vi "09-QNET_MECHKIT_Encoder.vi"() -> ()   [LabVIEW 2012]
doc: "This VI is to be used with the NI-ELVIS and the QNET-Mechatronic Sensors I module. The objective is learn about the behaviour of encoders."
uses:
  <vilib>/Simulation/Scripting/Companion Diagram/SimConfigNode/SimParams.ctl
  <vilib>/Simulation/Scripting/Companion Diagram/SimConfigNode/_simSolvers.ctl
  <vilib>/Simulation/Implementation/Shared/SIMSCR Execution Mode.ctl
  <vilib>/Simulation/Param Hierarchy/Typedefs/SIMPH Param Control Actions.ctl
  <vilib>/Simulation/Implementation/Shared/NILVSim_ParamChanged.vi
  <vilib>/Simulation/SignalDisplay/Implementation/NILVSim Time Waveform.llb/SIM Time Waveform (vector).vi
  <vilib>/Simulation/Utility/Implementation/SIM Halt.vi
  <vilib>/Simulation/SignalDisplay/Implementation/NILVSim Time Waveform.llb/SIM Time Waveform (scalar).vi
  <vilib>/Simulation/Implementation/Shared/NILVSim_Manager.vi
  <vilib>/Simulation/Implementation/Shared/NILVSim_FinalizeModel.vi
  <vilib>/Simulation/Implementation/Shared/SIM Unbundle Sim Info.vi
  <vilib>/Utility/error.llb/Clear Errors.vi
  <vilib>/Simulation/Implementation/Shared/NILVSim_GetModelError.vi
  <vilib>/Simulation/Implementation/Shared/SIM Bundle Sim Info.vi
  <vilib>/Simulation/Implementation/Shared/SIMSH Read Queue.vi
  <vilib>/Simulation/Implementation/Shared/NILVSim_Initialize.vi
  QNET Library/QNET_Drivers.llb/QNET_MECHKIT_AI_Read.vi
  <vilib>/Simulation/Utility/Implementation/NILVSim Get Time and IsAcceptedStep.vi
  <vilib>/Simulation/Scripting/Companion Diagram/SimConfigNode/SimDog.xnode
  QNET Library/QNET_MECHKIT_Functions/qnet_mechkit_decoder.vi
  <vilib>/Simulation/Implementation/XNodeFramework/SimXNode/SimX.xnode
  <vilib>/Simulation/Implementation/Shared/NI_SIM_Implementation.lvlib
panel:
  out "Encoder A and B (V)":waveform(dbl)[](graph)
  out "Encoder Index (V)":waveform(dbl)(graph)
  in  "Reset":bool
  in  "Enable Index":bool
  out "Angle (deg)":dbl
  out "16 bit Position (counts)":i16
  in  "Counts per rev":i16
  in  "Reload Value (counts)":i16
  in  "Sampling Rate (Hz)":dbl=100.0 min=0.0 max=1000.0 step=25.0 format="%.1f"
  in  "Device":tag="Dev1"
  in  "Stop":bool
  # "QNET-MECHKIT Encoder"
  # "NOTE: Place J7 to \"Enc A\", J8 to \"Enc B\", and J10 to \"Enc I\"."
  # "s"
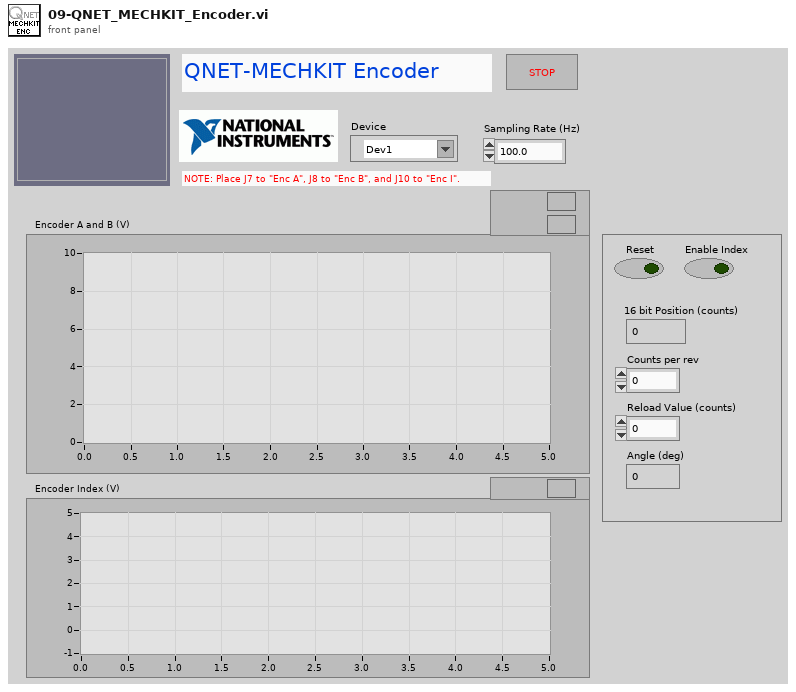
[diagram p1: front panel]
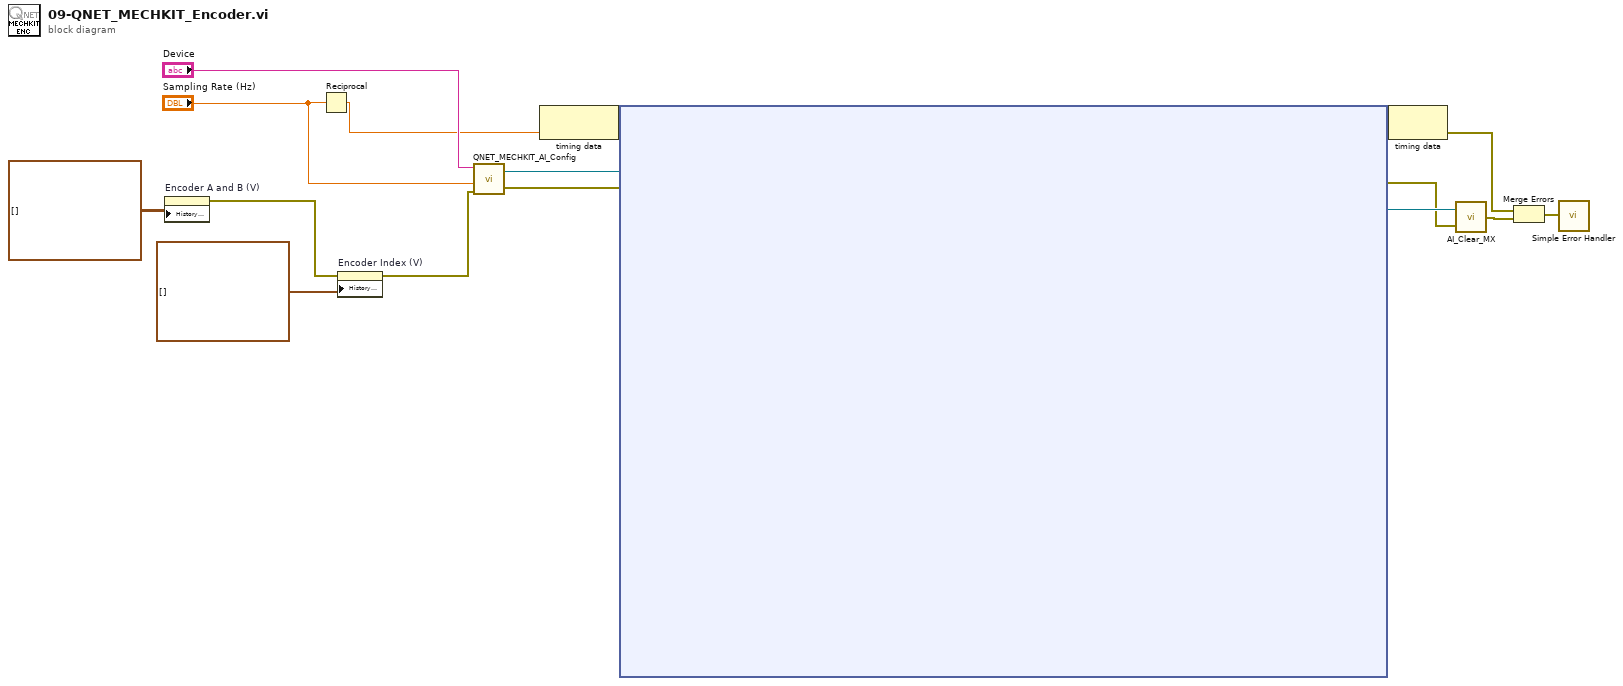
[diagram p0: block diagram]
diagram:
  n1 = property on="Encoder A and B (V)" class="WFChart (strict)"("History Data"=waveform(dbl)[][] []) -> (error out=w2:errorcluster)  [unwired: 2 in, 1 out]
  n2 = Reciprocal(x="Sampling Rate (Hz)") -> (1/x=w11:dbl)
  n3 = property on="Encoder Index (V)" class="WFChart (strict)"(error in=w2, "History Data"=waveform(dbl)[] []) -> (error out=w1:errorcluster)  [unwired: 1 in, 1 out]
  n4 = call "QNET_MECHKIT_AI_Config.vi"("error in"=w1, "sampling rate (Hz)"="Sampling Rate (Hz)", "dev"="Device") -> ("error out"=w10:errorcluster, "task out"=w16:refnum<k21>)  [unwired: 1 in]
  n5 = node-c288(w11) -> (w13:variant)
  n6 = node-c254 ("Simulation Loop")(w13, w16, w10) -> (w12:variant, w15:refnum<k21>, w9:errorcluster)
  n7 = node-c288(w12) -> (w7:errorcluster)
  n8 = call "AI_Clear_MX.vi"("Error in"=w9, "Task in"=w15) -> ("Error out"=w6:errorcluster)
  n9 = Merge Errors(w7, w6) -> (w5:errorcluster)
  n10 = call <vilib>:"Simple Error Handler.vi"("error in (no error)"=w5) -> ()  [unwired: 1 in, 8 out]
